vi "ADS1256 Example.vi"() -> ()   [LabVIEW 2020]
uses:
  ADS1256 ADC/Channel Selection.ctl
  <vilib>/MakerHub/LINX/Public/Peripherals/SPI/SPI CS Config.ctl
  <vilib>/MakerHub/LINX/Private/Type Defs/Peripherals/SPI/SPI CS Logic Level.ctl
  <vilib>/MakerHub/LINX/Private/Type Defs/Peripherals/SPI/SPI Configuration.ctl
  <vilib>/MakerHub/LINX/Private/Type Defs/Peripherals/SPI/SPI Bit Order.ctl
  <vilib>/MakerHub/LINX/Private/Type Defs/Peripherals/SPI/SPI Mode.ctl
  ADS1256 ADC/Programmable Gain Selection.ctl
  ADS1256 ADC/Sample Rate.ctl
  <vilib>/MakerHub/LINX/Public/Utilities/Open Local.vi
  LINX SPI/LINX SPI.lvclass
  ADS1256 ADC/LINX-ADS1256.lvclass
  <vilib>/MakerHub/LINX/LMH-LINX.lvlib
panel:
  in  "Channels":T1[](array[typedef])=[enum."Single Ended 0"]
  out "Waveform Chart":dbl[][](graph)
  in  "stop":bool
  out "Error Out":errorcluster
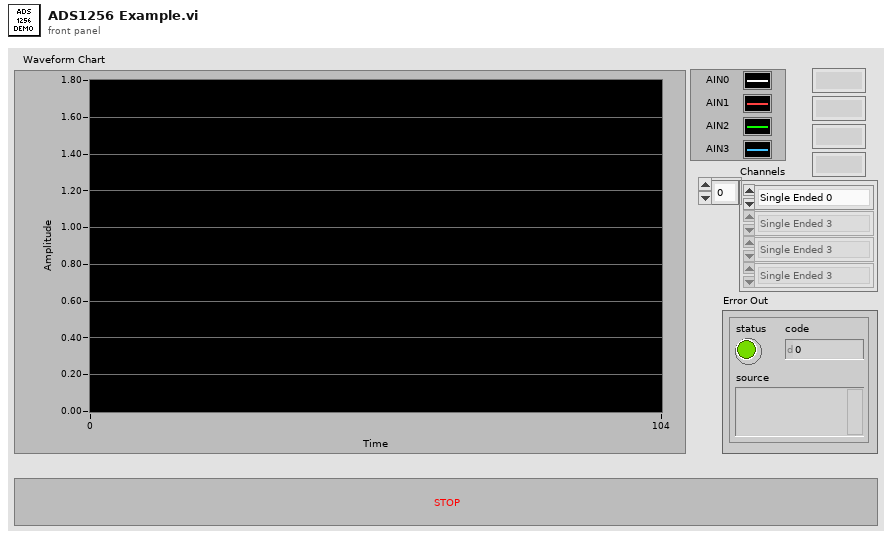
[diagram p1: front panel]
types:
  T1 = typedef "LINX-ADS1256.lvclass/Channel Selection.ctl" = enum16{"Differential 0-1", "Differential 2-3", "Differential 4-5", "Differential 6-7", "Single Ended 0", "Single Ended 1", "Single Ended 2", "Single Ended 3", "Single Ended 4", "Single Ended 5", "Single Ended 6", "Single Ended 7"}
  T2 = typedef "LINX-ADS1256.lvclass/Sample Rate.ctl" = enum16{"2.5Hz", "5Hz", "10Hz", "15Hz", "25Hz", "30Hz", "50Hz", "60Hz", "100Hz", "500Hz", "1000Hz", "2000Hz", "3750Hz", "7500Hz", "15000Hz", "30000Hz"}
  T3 = typedef "LINX-ADS1256.lvclass/Programmable Gain Selection.ctl" = enum16{"+/-5V (1)", "+/-2.5V (2)", "+/-1.25V (4)", "+/-0.625V (8)", "+/-312.5mV (16)", "+/-156.25mV (32)", "+/-78.125mV (64)"}
  T4 = typedef "LMH-LINX.lvlib/SPI Configuration.ctl" = cluster{"Clock Frequency":u32, "Bit Order":T5, "SPI Mode":T6}
  T5 = typedef "LMH-LINX.lvlib/SPI Bit Order.ctl" = enum8{"LSb First", "MSb First"}
  T6 = typedef "LMH-LINX.lvlib/SPI Mode.ctl" = enum8{"Mode 0", "Mode 1", "Mode 2", "Mode 3"}
  T7 = typedef "LMH-LINX.lvlib/SPI CS Config.ctl" = cluster{"CS Channel":u8, "CS Logic Level":T8}
  T8 = typedef "LMH-LINX.lvlib/SPI CS Logic Level.ctl" = enum8{"Active Low", "Active High"}
  T9 = typedef "LMH-LINX.lvlib/LINX Ref.ctl" = cluster{"IO":T10, "Interface":T11, "LINX Device Config":T12}
  T10 = typedef "LMH-LINX.lvlib/Platform.ctl" = enum16{"Remote", "Local"}
  T11 = typedef "LMH-LINX.lvlib/Interface.ctl" = enum16{"Serial", "TCP"}
  T12 = typedef "LMH-LINX.lvlib/Device.lvlib/LINX Device Config.ctl" = cluster{"Interface":T11, "COM Port":refnum<visa-resource-name>, "TCP Configuration":T13, "Device Family":u8, "Device ID":u8, "Device Name":string, "TCP Ref":refnum<k5>, "Channels":T14}
  T13 = typedef "LMH-LINX.lvlib/Device.lvlib/TCP Config.ctl" = cluster{"IP Address":string, "Port":u16}
  T14 = typedef "LMH-LINX.lvlib/Channels.ctl" = cluster{"DI":u8[], "DO":u8[], "AI":u8[], "AO":u8[], "PWM":u8[], "QE":u8[], "UART":u8[], "I2C 2":u8[], "SPI":u8[], "CAN":u8[], "Servo":u8[], "AI Ref (V)":dbl, "AI Resolution (Bits)":u8, "AO Ref (V)":dbl, "AO Resolution (Bits)":u8}
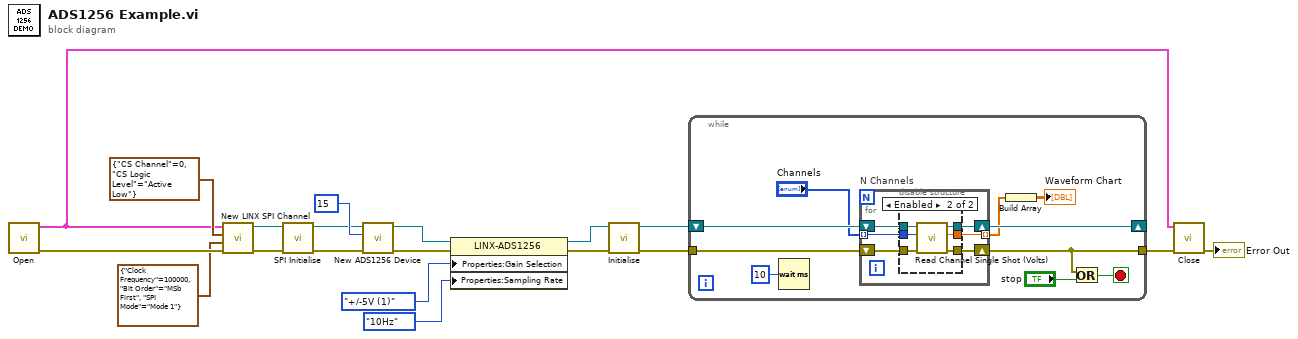
[diagram p0: block diagram]
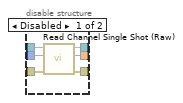
[diagram p2: hidden frame]
diagram:
  n1 = call-poly <vilib>:"Open.vi"() -> ("Error Out"=w17:errorcluster, "LINX Resource"=w11:T9)  [unwired: 9 in, 1 out]
  n2 = call "New LINX SPI Channel.vi"("error in (no error)"=w17, "SPI Configuration"=T4 {"Clock Frequency"=100000, "Bit Order"=enum."MSb First", "SPI Mode"=enum."Mode 1"}, "CS Configuration"=T7 {"CS Channel"=0, "CS Logic Level"=enum."Active Low"}, "LINX Resource"=w11) -> ("error out"=w14:errorcluster, "LINX SPI out"=w15:refnum<class "LINX SPI.lvclass">)  [unwired: 6 in]
  n3 = call-dynamic "SPI Initialise.vi"("error in (no error)"=w14, "LINX SPI in"=w15) -> ("error out"=w12:errorcluster, "LINX SPI out"=w13:refnum<class "LINX SPI.lvclass">)  [unwired: 8 in]
  n4 = call "New ADS1256 Device.vi"("error in (no error)"=w12, "SPI CS Line"=u8 15 ("I2C Slave Address (0x48)"), "SPI"=w13) -> ("error out"=w9:errorcluster, "LINX-ADS1X15 out"=w5:refnum<class "LINX-ADS1256.lvclass">)  [unwired: 7 in]
  n5 = property class="LINX-ADS1256"(reference=w5, error in=w9, "Properties:Gain Selection"=Programmable_Gain_Selection."+/-5V (1)" ("Gain Selection"), "Properties:Sampling Rate"=Sample_Rate."10Hz" ("Sampling Rate")) -> (reference out=w4:refnum<class "LINX-ADS1256.lvclass">, error out=w6:errorcluster)
  n6 = call "Initialise.vi"("error in (no error)"=w6, "LINX-ADS1256 in"=w4) -> ("error out"=w7:errorcluster, "LINX-ADS1256 out"=w8:refnum<class "LINX-ADS1256.lvclass">)  [unwired: 8 in]
  n7 = while {
    tunnel: w7 -> [w28]
    shift-right: [w24] -> _
    shift-left: w8 -> [w29]
    tunnel: [w23] -> w1
    stop <- w25 stop-if-true
    n8 = Wait (ms)(milliseconds to wait=u32 10) -> ()  [unwired: 1 out]
    n9 = for "N Channels" {
      tunnel: "Channels" -> [w33] mode=indexing
      tunnel: [w30] -> w22 mode=indexing
      shift-right: [w32] -> w24
      shift-left: w29 -> [w35]
      shift-right: [w31] -> w23
      shift-left: w28 -> [w34]
      n10 = disable-structure shown="Enabled" {
        disable-tunnel: w35 -> [w41 w47]
        disable-tunnel: w34 -> [w39 w45]
        disable-tunnel: w33 -> [w37 w46]
        disable-tunnel: [w40 w44] -> w32
        disable-tunnel: [w38 w42] -> w31
        disable-tunnel: [w36 w43] -> w30
        frame Disabled {
          n11 = call "Read Channel Single Shot (Raw).vi"("error in (no error)"=w39, "ADC Channel Selection"=w37, "LINX-ADS1256 in"=w41) -> ("error out"=w38:errorcluster, "ADC Raw"=w36:i32, "LINX-ADS1256 out"=w40:refnum<class "LINX-ADS1256.lvclass">)  [unwired: 6 in]
        }
        frame Enabled {
          n12 = call "Read Channel Single Shot (Volts).vi"("error in (no error)"=w45, "ADC Channel Selection"=w46, "LINX-ADS1256 in"=w47) -> ("error out"=w42:errorcluster, "ADC Volts"=w43:dbl, "LINX-ADS1256 out"=w44:refnum<class "LINX-ADS1256.lvclass">)  [unwired: 6 in]
        }
      }
    }
    n13 = Build Array(w22) -> (→"Waveform Chart":dbl[][])
    n14 = Or(x=w23, y="stop") -> (x .or. y?=w25:bool)
  }
  n15 = call <vilib>:"Close.vi"("Error In"=w1, "LINX Resource"=w11) -> ("Error Out"=→"Error Out":errorcluster)  [unwired: 9 in]
